vi "decode_spinningdisk_querystr.vi"(0 "input string":string, 3 "error in":errorcluster) -> (4 "shutter":bool, 5 "disk spinning":bool, 6 "disk position":bool, 7 "excitation filter":u16, 8 "emission filter":u16, 9 "dichroic mirror":u16, 10 "error out":errorcluster)   [LabVIEW 2016]
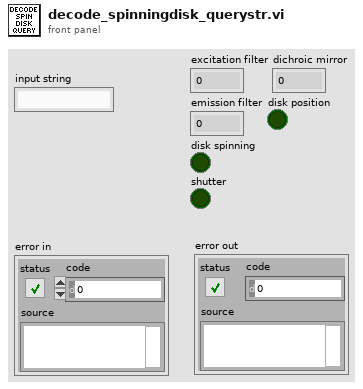
[diagram p1: front panel]
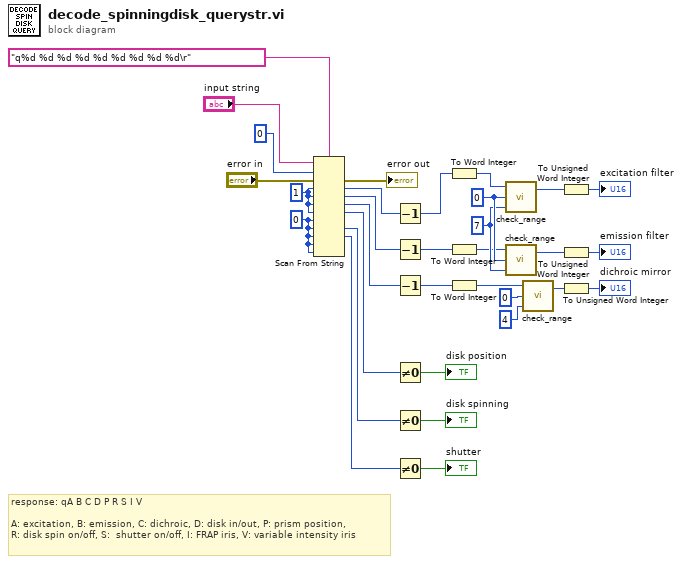
[diagram p0: block diagram]
diagram:
  w13 = i16 7 ("max")
  w14 = i16 0 ("min")
  w17 = 0 ("default value 5")
  w30 = 1 ("default value 1")
  # "response: qA B C D P R S I V\n\nA: excitation, B: emission, C: dichroic, D: disk in/out, P: prism position, \nR: disk spin on/off, S:  shutter on/off, I: FRAP iris, V: variable intensity iris"
  n1 = Scan From String(format string="q%d %d %d %d %d %d %d %d %d\r", input string="input string", initial scan location=u32 0, error in="error in", default 1=w30, default 2=w30, default 3=w30, default 4=w30, default 5=w17, default 6=w17, default 7=w17, default 8=w17, default 9=w17) -> (error out=→"error out":errorcluster, output 1=w29:i32, output 2=w28:i32, output 3=w27:i32, output 4=w25:i32, output 6=w26:i32, output 7=w24:i32)  [unwired: 3 in, 2 out]
  n2 = Decrement(x=w29) -> (x-1=w16:i32)
  n3 = Decrement(x=w28) -> (x-1=w12:i32)
  n4 = Decrement(x=w27) -> (x-1=w10:i32)
  n5 = Not Equal To 0?(x=w25) -> (x != 0?=→"disk position":bool)
  n6 = Not Equal To 0?(x=w26) -> (x != 0?=→"disk spinning":bool)
  n7 = Not Equal To 0?(x=w24) -> (x != 0?=→"shutter":bool)
  n8 = To Word Integer(number=w16) -> (16bit integer=w6:i16)
  n9 = To Word Integer(number=w12) -> (16bit integer=w5:i16)
  n10 = To Word Integer(number=w10) -> (16bit integer=w4:i16)
  n11 = call "check_range.vi"("max"=w13, "min"=w14, "x"=w6) -> ("checked x"=w15:i16)  [unwired: 1 in]
  n12 = call "check_range.vi"("max"=w13, "min"=w14, "x"=w5) -> ("checked x"=w11:i16)  [unwired: 1 in]
  n13 = call "check_range.vi"("max"=i16 4, "min"=i16 0, "x"=w4) -> ("checked x"=w7:i16)  [unwired: 1 in]
  n14 = To Unsigned Word Integer(number=w15) -> (unsigned 16bit integer=→"excitation filter":u16)
  n15 = To Unsigned Word Integer(number=w11) -> (unsigned 16bit integer=→"emission filter":u16)
  n16 = To Unsigned Word Integer(number=w7) -> (unsigned 16bit integer=→"dichroic mirror":u16)
